vi "Move new property node.vi"(8 "error in":errorcluster, 9 "New objects created":refnum<vi>[](array[refnum]), 10 "Property Node Ref":refnum<vi>, 11 "Terminal Data Cluster":T1) -> (0 "error out":errorcluster)   [LabVIEW 2023]
doc: "Because a bundler will expand to the right once its labels are set, and we want to place the bundler to the left of a sink terminal, this VI will adjust the new objects created (a bundler and optional constant) to be posisioned the correct offset from the affected terminal. Offset is by default -15px.\n\nThis is not needed for bundlers on source terminals, so we ignore those."
panel:
  out "Move":i32
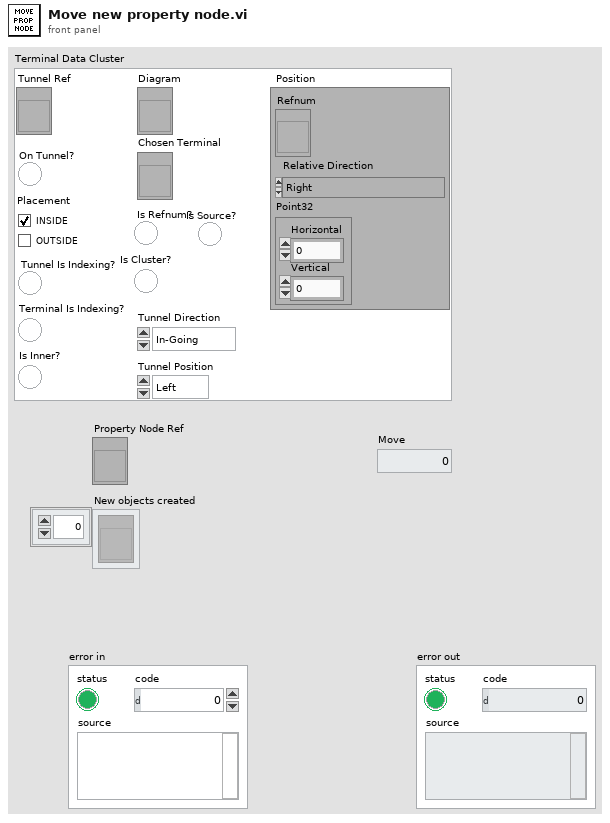
[diagram p1: front panel]
types:
  T1 = cluster{"Tunnel Ref":refnum<vi>, "On Tunnel?":bool, "Placement":enum32{"Choice 1", "Choice 2"}, "Tunnel Is Indexing?":bool, "Diagram":refnum<vi>, "Position":cluster{"Refnum":refnum<vi>, "Relative Direction":enum32{"Right", "Left", "Top", "Bottom", "Top Right", "Top Left", "Bottom Right", "Bottom Left"}, "Point32":cluster{"Horizontal":i32, "Vertical":i32}}, "Chosen Terminal":refnum<vi>, "Is Refnum?":bool, "Is Cluster?":bool, "Is Source?":bool, "Tunnel Direction":enum16{"In-Going", "Out-Going"}, "Tunnel Position":enum16{"Left", "Top", "Right", "Bottom"}, "Is Inner?":bool, "Terminal Is Indexing?":bool}
  T2 = typedef "LVRectTypeDef.ctl" = cluster{"Left":i16, "Top":i16, "Right":i16, "Bottom":i16}
  T3 = typedef "LVPositionTypeDef.ctl" = cluster{"Left":i32, "Top":i32}
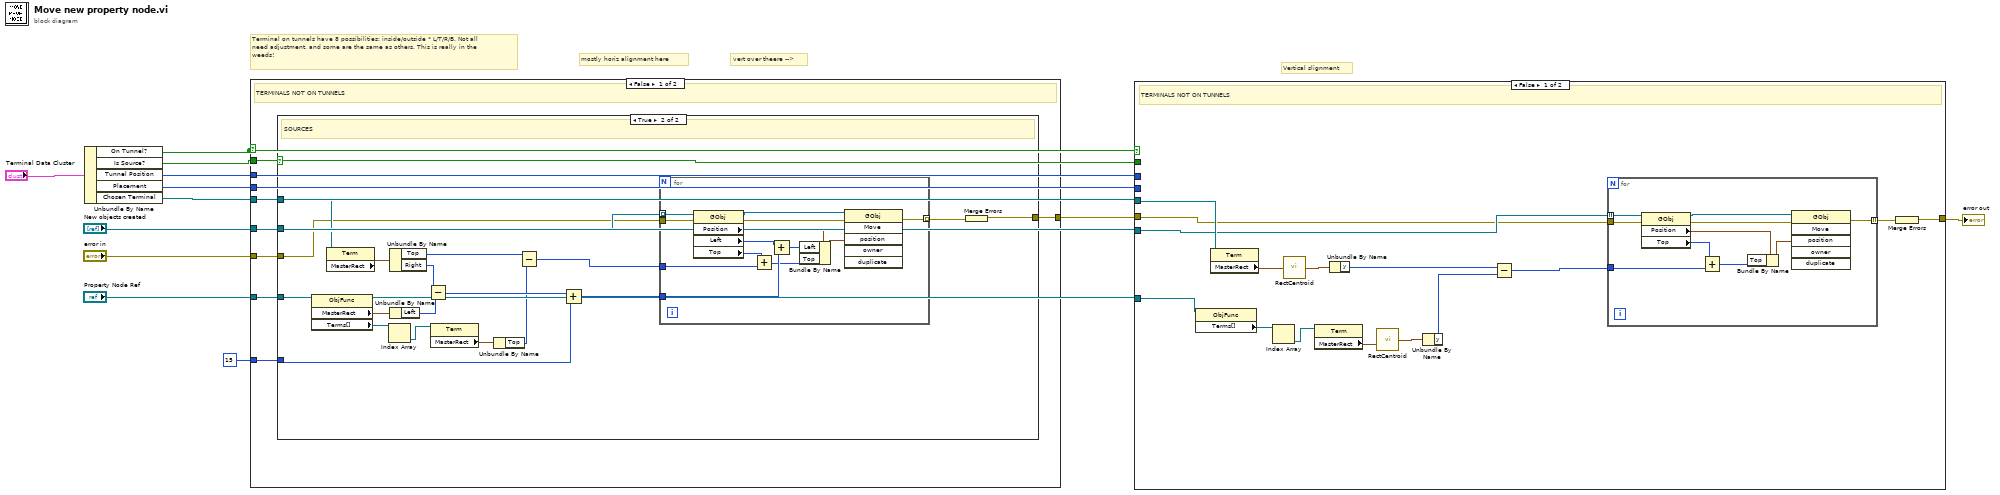
[diagram p0: block diagram]
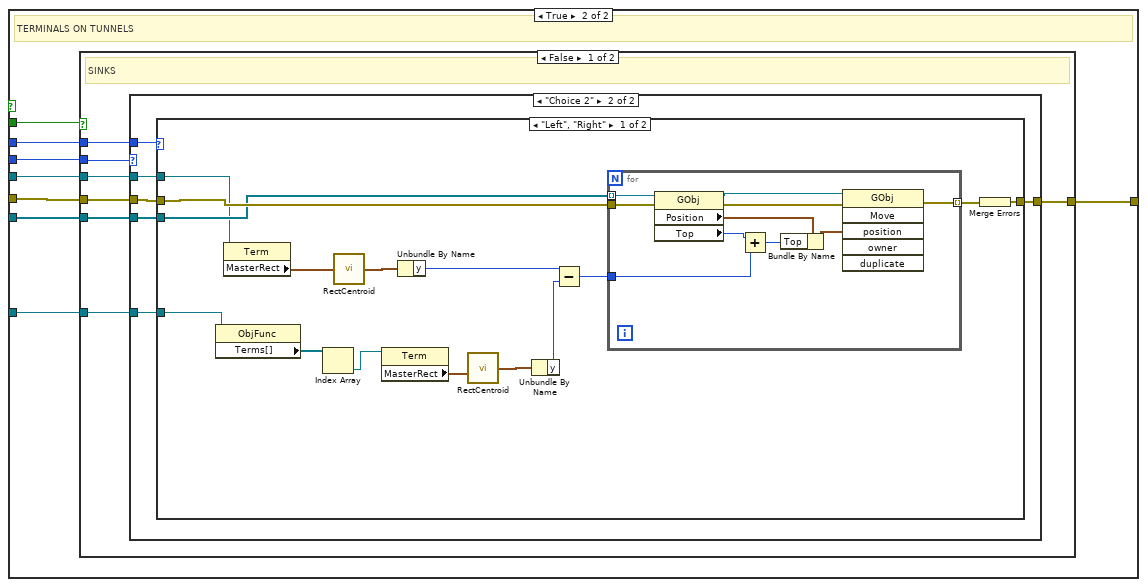
[diagram p2: hidden frame]
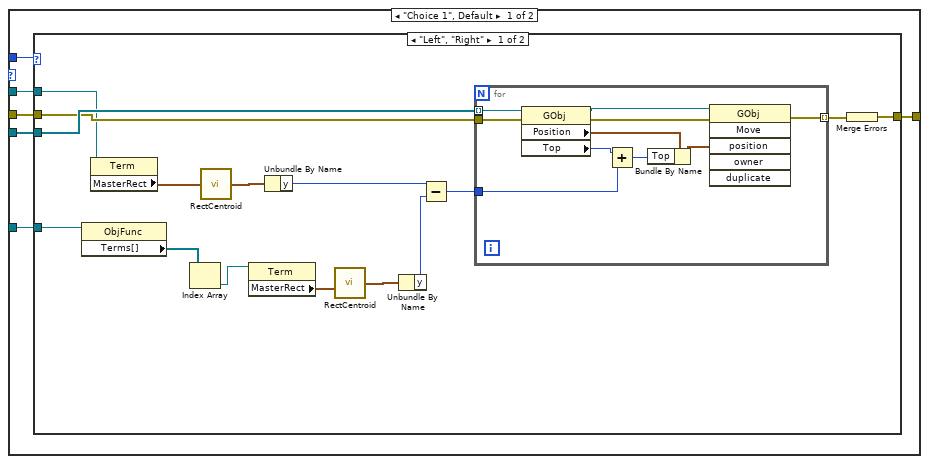
[diagram p3: hidden frame]
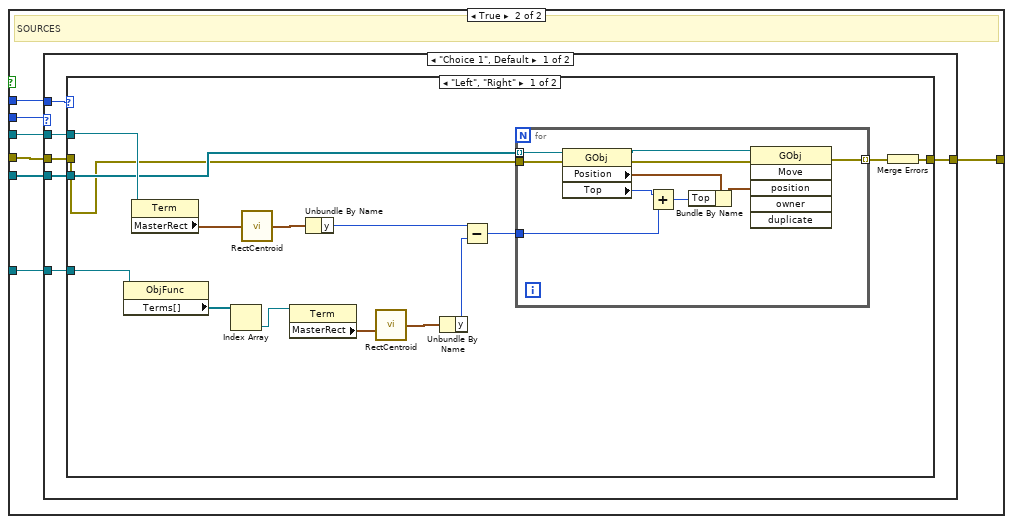
[diagram p6: hidden frame]
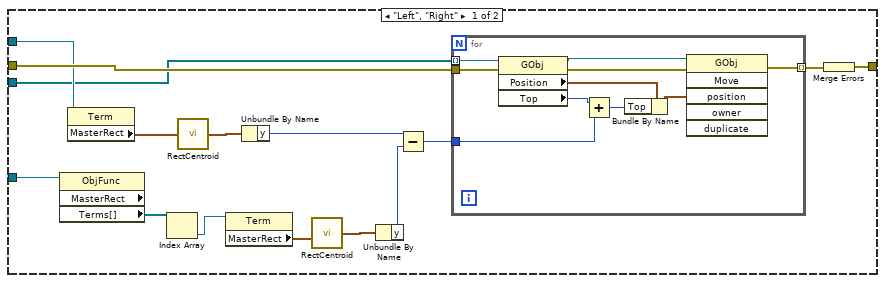
[diagram p9: hidden frame]
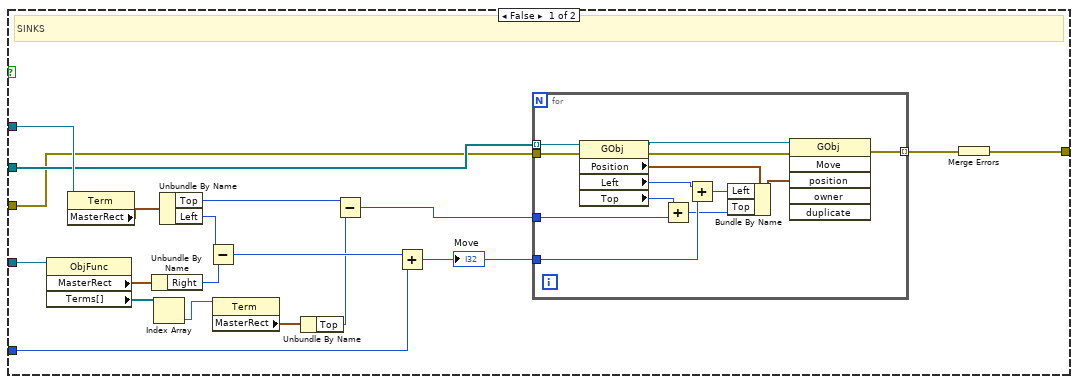
[diagram p10: hidden frame]
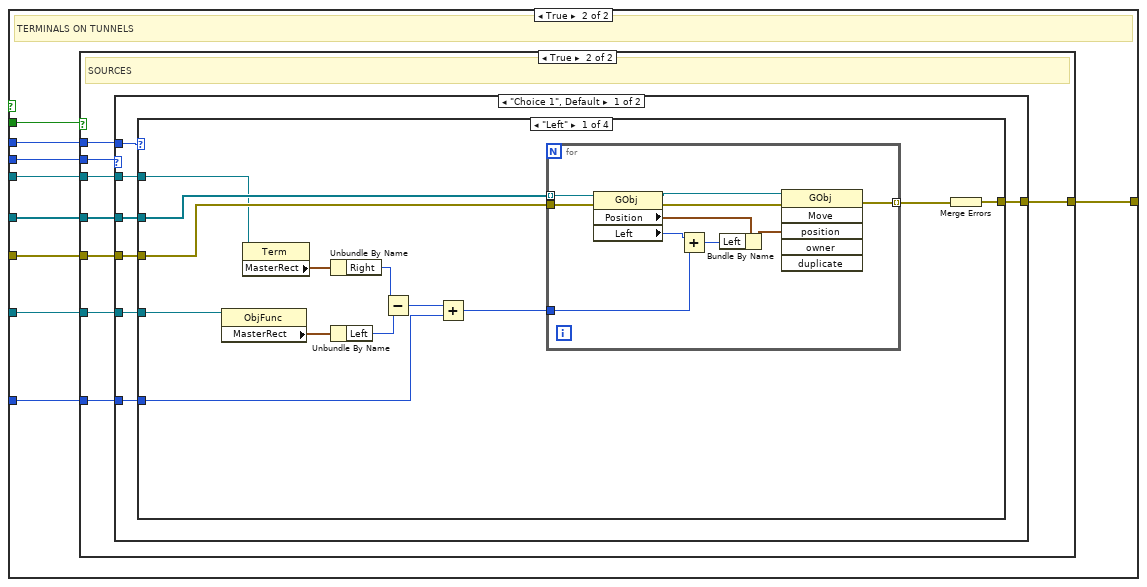
[diagram p11: hidden frame]
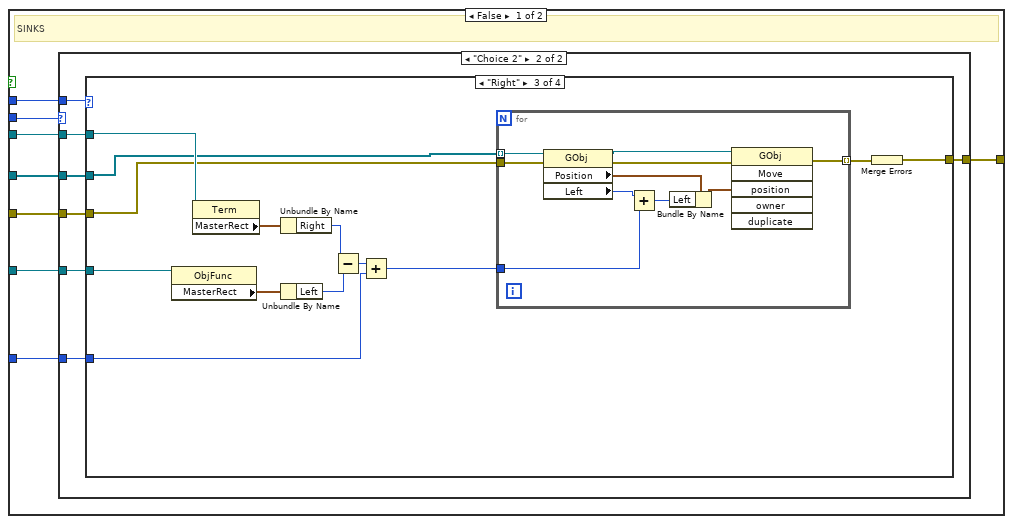
[diagram p12: hidden frame]
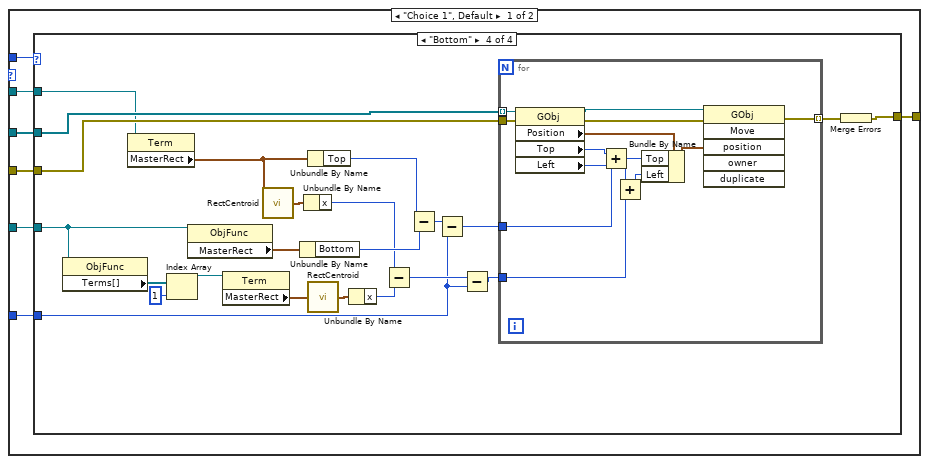
[diagram p13: hidden frame]
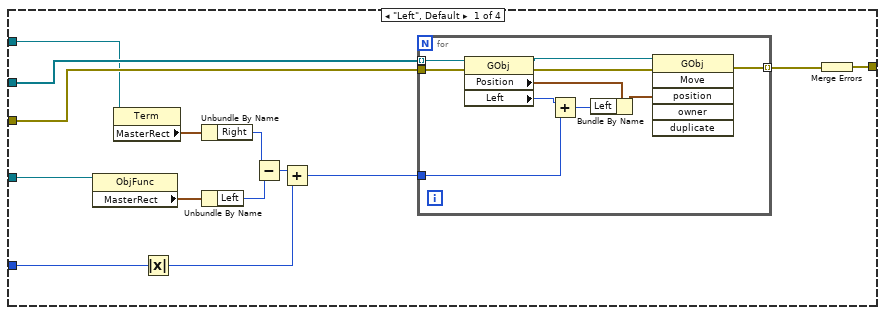
[diagram p14: hidden frame]
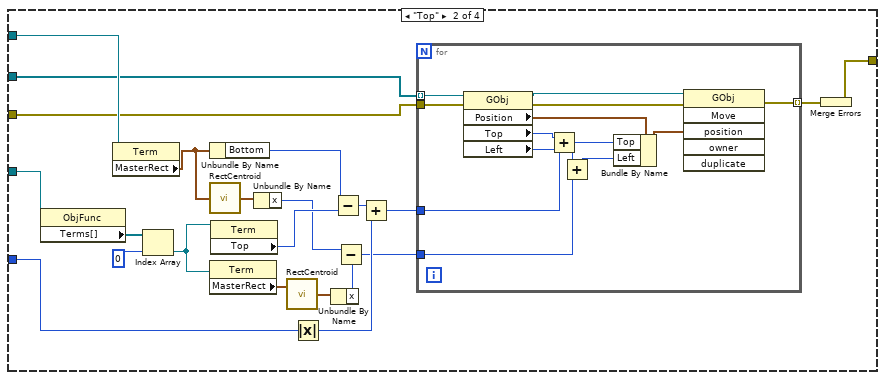
[diagram p15: hidden frame]
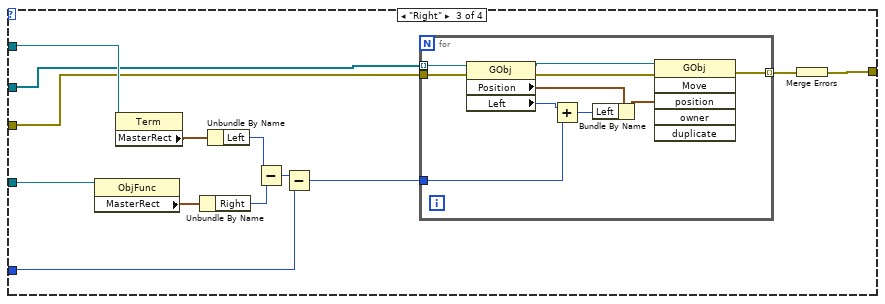
[diagram p16: hidden frame]
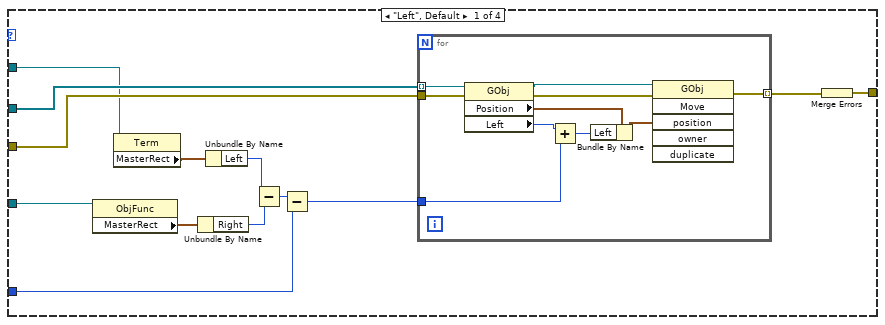
[diagram p17: hidden frame]
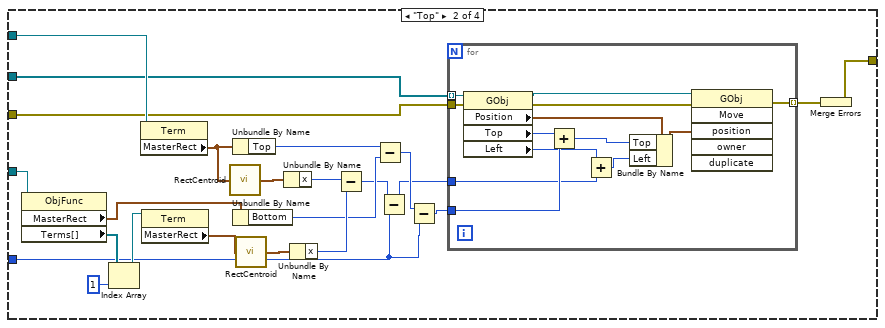
[diagram p18: hidden frame]
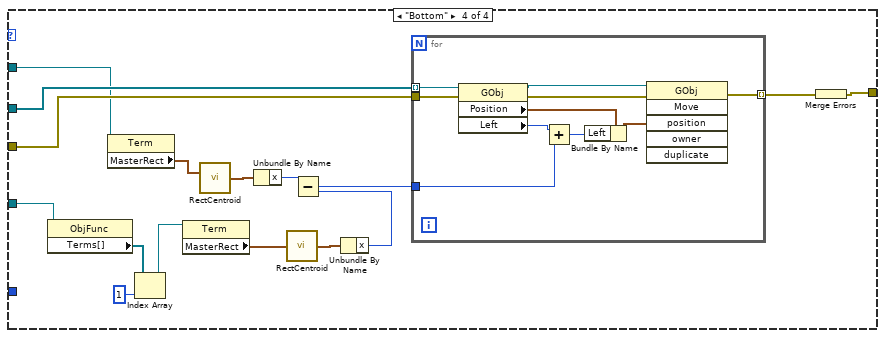
[diagram p19: hidden frame]
diagram:
  # "vert over theere -->"
  # "mostly horiz alignment here"
  # "Vertical slignment"
  # "Terminal on tunnels have 8 possibilities: inside/outside * L/T/R/B. Not all need adjustment, and some are the same as others. This is really in the weeds!"
  n1 = Unbundle By Name("Terminal Data Cluster") -> ("On Tunnel?"=w7:bool, "Is Source?"=w10:bool, "Tunnel Position"=w6:enum16{"Left", "Top", "Right", "Bottom"}, "Placement"=w5:enum32{"Choice 1", "Choice 2"}, "Chosen Terminal"=w4:refnum<vi>)
  n2 = case shown="False" w7 {
    tunnel: 15 ("Offset") -> [w13 w84]
    tunnel: "Property Node Ref" -> [w14 w86]
    tunnel: [w19 w89] -> w9
    tunnel: "error in" -> [w17 w88]
    tunnel: w10 -> [w18 w92]
    tunnel: w4 -> [w16 w85]
    tunnel: w6 -> [_ w91]
    tunnel: w5 -> [_ w90]
    tunnel: "New objects created" -> [w15 w87]
    frame False {
      # "TERMINALS NOT ON TUNNELS"
      n3 = case shown="True" w18 {
        tunnel: w13 -> [w37 w53]
        tunnel: w14 -> [w36 w54]
        tunnel: w16 -> [w34 w55]
        tunnel: [w28 w57] -> w19
        tunnel: w15 -> [w27 w56]
        tunnel: w17 -> [w26 w52]
        frame False {
          # "SINKS"
          n4 = property class="ObjFunc"(reference=w36) -> ("MasterRect"=w35:T2, "Terms[]"=w25:refnum<vi>[])  [unwired: 1 in, 2 out]
          n5 = property class="Term"(reference=w34) -> ("MasterRect"=w33:T2)  [unwired: 1 in, 2 out]
          n6 = Unbundle By Name(w35) -> ("Right"=w31:i16)
          n7 = Index Array(array=w25) -> (element=w24:refnum<vi>)  [unwired: 1 in]
          n8 = Unbundle By Name(w33) -> ("Top"=w22:i16, "Left"=w32:i16)
          n9 = Subtract(x=w32, y=w31) -> (x-y=w38:i16)
          n10 = property class="Term"(reference=w24) -> ("MasterRect"=w23:T2)  [unwired: 1 in, 2 out]
          n11 = Unbundle By Name(w23) -> ("Top"=w21:i16)
          n12 = Subtract(x=w22, y=w21) -> (x-y=w20:i16)
          n13 = Add(x=w38, y=w37) -> (x+y=w30:i32)
          "Move" <- w30
          n14 = for {
            tunnel: w27 -> [w51] mode=indexing
            tunnel: w30 -> [w48]
            tunnel: w26 -> [w44]
            tunnel: [w42] -> w29 mode=indexing
            tunnel: w20 -> [w40]
            n15 = property class="GObj"(reference=w51, error in=w44) -> (reference out=w50:refnum<vi>, error out=w43:errorcluster, "Position"=w47:T3, "Left"=w49:i32, "Top"=w41:i32)
            n16 = Add(x=w41, y=w40) -> (x+y=w39:i32)
            n17 = Add(x=w49, y=w48) -> (x+y=w46:i32)
            n18 = Bundle By Name(cluster=w47, "Left"=w46, "Top"=w39) -> (w45:T3)
            n19 = invoke class="GObj" method="Move"(reference=w50, error in=w43, "position"=w45) -> (error out=w42:errorcluster)  [unwired: 3 in, 5 out]
          }
          n20 = Merge Errors(w29) -> (w28:errorcluster)
        }
        frame True {
          # "SOURCES"
          n21 = property class="ObjFunc"(reference=w54) -> ("MasterRect"=w69:T2, "Terms[]"=w63:refnum<vi>[])  [unwired: 1 in, 2 out]
          n22 = property class="Term"(reference=w55) -> ("MasterRect"=w68:T2)  [unwired: 1 in, 2 out]
          n23 = Index Array(array=w63) -> (element=w62:refnum<vi>)  [unwired: 1 in]
          n24 = Unbundle By Name(w68) -> ("Top"=w60:i16, "Right"=w67:i16)
          n25 = Unbundle By Name(w69) -> ("Left"=w66:i16)
          n26 = Subtract(x=w67, y=w66) -> (x-y=w70:i16)
          n27 = property class="Term"(reference=w62) -> ("MasterRect"=w61:T2)  [unwired: 1 in, 2 out]
          n28 = Unbundle By Name(w61) -> ("Top"=w59:i16)
          n29 = Subtract(x=w60, y=w59) -> (x-y=w58:i16)
          n30 = Add(x=w70, y=w53) -> (x+y=w65:i32)
          n31 = for {
            tunnel: w56 -> [w83] mode=indexing
            tunnel: w65 -> [w80]
            tunnel: w52 -> [w76]
            tunnel: [w74] -> w64 mode=indexing
            tunnel: w58 -> [w72]
            n32 = property class="GObj"(reference=w83, error in=w76) -> (reference out=w82:refnum<vi>, error out=w75:errorcluster, "Position"=w79:T3, "Left"=w81:i32, "Top"=w73:i32)
            n33 = Add(x=w73, y=w72) -> (x+y=w71:i32)
            n34 = Add(x=w81, y=w80) -> (x+y=w78:i32)
            n35 = Bundle By Name(cluster=w79, "Left"=w78, "Top"=w71) -> (w77:T3)
            n36 = invoke class="GObj" method="Move"(reference=w82, error in=w75, "position"=w77) -> (error out=w74:errorcluster)  [unwired: 3 in, 5 out]
          }
          n37 = Merge Errors(w64) -> (w57:errorcluster)
        }
      }
    }
    frame True {
      # "TERMINALS ON TUNNELS"
      n38 = case shown="True" w92 {
        tunnel: w91 -> [w100 w348]
        tunnel: w90 -> [w99 w347]
        tunnel: [w98 w341] -> w89
        tunnel: w88 -> [w97 w344]
        tunnel: w87 -> [w96 w345]
        tunnel: w86 -> [w95 w343]
        tunnel: w85 -> [w94 w346]
        tunnel: w84 -> [w93 w342]
        frame False {
          # "SINKS"
          n39 = case shown="\"Choice 2\"" w99 {
            tunnel: w100 -> [w107 w232]
            tunnel: [w101 w231] -> w98
            tunnel: w97 -> [w104 w230]
            tunnel: w96 -> [w105 w229]
            tunnel: w95 -> [w102 w228]
            tunnel: w94 -> [w106 w227]
            tunnel: w93 -> [w103 w226]
            frame "Choice 1", Default {
              n40 = case shown="\"Bottom\"" w107 {
                tunnel: [w116 w147 w179 w203] -> w101
                tunnel: w104 -> [w120 w149 w176 w205]
                tunnel: w105 -> [w121 w148 w177 w206]
                tunnel: w102 -> [w119 w146 w175 w202]
                tunnel: w106 -> [w118 w150 w178 w204]
                tunnel: w103 -> [w117 w142 w174 w192]
                frame "Left", Default {
                  n41 = property class="ObjFunc"(reference=w119) -> ("MasterRect"=w114:T2)  [unwired: 1 in, 2 out]
                  n42 = property class="Term"(reference=w118) -> ("MasterRect"=w113:T2)  [unwired: 1 in, 2 out]
                  n43 = Absolute Value(x=w117) -> (abs(x)=w108:i32)
                  n44 = Unbundle By Name(w113) -> ("Right"=w112:i16)
                  n45 = Unbundle By Name(w114) -> ("Left"=w111:i16)
                  n46 = Subtract(x=w112, y=w111) -> (x-y=w115:i16)
                  n47 = Add(x=w115, y=w108) -> (x+y=w110:i32)
                  n48 = for {
                    tunnel: w110 -> [w129]
                    tunnel: [w124] -> w109 mode=indexing
                    tunnel: w121 -> [w123] mode=indexing
                    tunnel: w120 -> [w122]
                    n49 = property class="GObj"(reference=w123, error in=w122) -> (reference out=w131:refnum<vi>, error out=w125:errorcluster, "Position"=w128:T3, "Left"=w130:i32)
                    n50 = Add(x=w130, y=w129) -> (x+y=w127:i32)
                    n51 = Bundle By Name(cluster=w128, "Left"=w127) -> (w126:T3)
                    n52 = invoke class="GObj" method="Move"(reference=w131, error in=w125, "position"=w126) -> (error out=w124:errorcluster)  [unwired: 3 in, 5 out]
                  }
                  n53 = Merge Errors(w109) -> (w116:errorcluster)
                }
                frame "Top" {
                  n54 = property class="ObjFunc"(reference=w146) -> ("Terms[]"=w145:refnum<vi>[])  [unwired: 1 in, 2 out]
                  n55 = property class="Term"(reference=w150) -> ("MasterRect"=w137:T2)  [unwired: 1 in, 2 out]
                  n56 = Index Array(array=w145, index=0) -> (element=w138:refnum<vi>)
                  n57 = Unbundle By Name(w137) -> ("Bottom"=w140:i16)
                  n58 = call <vilib>:"RectCentroid.vi"("rect"=w137) -> ("point"=w136:cluster{"x":i16, "y":i16})
                  n59 = property class="Term"(reference=w138) -> ("MasterRect"=w133:T2)  [unwired: 1 in, 2 out]
                  n60 = property class="Term"(reference=w138) -> ("Top"=w144:i32)  [unwired: 1 in, 2 out]
                  n61 = Unbundle By Name(w136) -> ("x"=w135:i16)
                  n62 = call <vilib>:"RectCentroid.vi"("rect"=w133) -> ("point"=w134:cluster{"x":i16, "y":i16})
                  n63 = Absolute Value(x=w142) -> (abs(x)=w143:i32)
                  n64 = Unbundle By Name(w134) -> ("x"=w132:i16)
                  n65 = Subtract(x=w140, y=w144) -> (x-y=w153:i32)
                  n66 = Subtract(x=w135, y=w132) -> (x-y=w141:i16)
                  n67 = Add(x=w153, y=w143) -> (x+y=w152:i32)
                  n68 = for {
                    tunnel: w152 -> [w164]
                    tunnel: [w159] -> w151 mode=indexing
                    tunnel: w149 -> [w158]
                    tunnel: w148 -> [w157] mode=indexing
                    tunnel: w141 -> [w155]
                    n69 = property class="GObj"(reference=w157, error in=w158) -> (reference out=w166:refnum<vi>, error out=w160:errorcluster, "Position"=w163:T3, "Top"=w165:i32, "Left"=w156:i32)
                    n70 = Add(x=w165, y=w164) -> (x+y=w162:i32)
                    n71 = Add(x=w156, y=w155) -> (x+y=w154:i32)
                    n72 = Bundle By Name(cluster=w163, "Top"=w162, "Left"=w154) -> (w161:T3)
                    n73 = invoke class="GObj" method="Move"(reference=w166, error in=w160, "position"=w161) -> (error out=w159:errorcluster)  [unwired: 3 in, 5 out]
                  }
                  n74 = Merge Errors(w151) -> (w147:errorcluster)
                }
                frame "Right" {
                  n75 = property class="ObjFunc"(reference=w175) -> ("MasterRect"=w172:T2)  [unwired: 1 in, 2 out]
                  n76 = property class="Term"(reference=w178) -> ("MasterRect"=w171:T2)  [unwired: 1 in, 2 out]
                  n77 = Unbundle By Name(w172) -> ("Right"=w169:i16)
                  n78 = Unbundle By Name(w171) -> ("Left"=w170:i16)
                  n79 = Subtract(x=w170, y=w169) -> (x-y=w173:i16)
                  n80 = Subtract(x=w173, y=w174) -> (x-y=w168:i32)
                  n81 = for {
                    tunnel: w177 -> [w189] mode=indexing
                    tunnel: w168 -> [w186]
                    tunnel: w176 -> [w182]
                    tunnel: [w180] -> w167 mode=indexing
                    n82 = property class="GObj"(reference=w189, error in=w182) -> (reference out=w188:refnum<vi>, error out=w181:errorcluster, "Position"=w185:T3, "Left"=w187:i32)
                    n83 = Add(x=w187, y=w186) -> (x+y=w184:i32)
                    n84 = Bundle By Name(cluster=w185, "Left"=w184) -> (w183:T3)
                    n85 = invoke class="GObj" method="Move"(reference=w188, error in=w181, "position"=w183) -> (error out=w180:errorcluster)  [unwired: 3 in, 5 out]
                  }
                  n86 = Merge Errors(w167) -> (w179:errorcluster)
                }
                frame "Bottom" {
                  n87 = property class="ObjFunc"(reference=w202) -> ("Terms[]"=w201:refnum<vi>[])  [unwired: 1 in, 2 out]
                  n88 = property class="Term"(reference=w204) -> ("MasterRect"=w195:T2)  [unwired: 1 in, 2 out]
                  n89 = Index Array(array=w201, index=1) -> (element=w200:refnum<vi>)
                  n90 = property class="ObjFunc"(reference=w202) -> ("MasterRect"=w211:T2)  [unwired: 1 in, 2 out]
                  n91 = property class="Term"(reference=w200) -> ("MasterRect"=w199:T2)  [unwired: 1 in, 2 out]
                  n92 = call <vilib>:"RectCentroid.vi"("rect"=w195) -> ("point"=w196:cluster{"x":i16, "y":i16})
                  n93 = Unbundle By Name(w211) -> ("Bottom"=w209:i16)
                  n94 = Unbundle By Name(w196) -> ("x"=w194:i16)
                  n95 = Unbundle By Name(w195) -> ("Top"=w210:i16)
                  n96 = call <vilib>:"RectCentroid.vi"("rect"=w199) -> ("point"=w198:cluster{"x":i16, "y":i16})
                  n97 = Unbundle By Name(w198) -> ("x"=w197:i16)
                  n98 = Subtract(x=w194, y=w197) -> (x-y=w193:i16)
                  n99 = Subtract(x=w210, y=w209) -> (x-y=w212:i16)
                  n100 = Subtract(x=w212, y=w192) -> (x-y=w208:i32)
                  n101 = Subtract(x=w193, y=w192) -> (x-y=w191:i32)
                  n102 = for {
                    tunnel: w206 -> [w225] mode=indexing
                    tunnel: w208 -> [w222]
                    tunnel: w205 -> [w218]
                    tunnel: [w216] -> w207 mode=indexing
                    tunnel: w191 -> [w214]
                    n103 = property class="GObj"(reference=w225, error in=w218) -> (reference out=w224:refnum<vi>, error out=w217:errorcluster, "Position"=w221:T3, "Top"=w223:i32, "Left"=w215:i32)
                    n104 = Add(x=w223, y=w222) -> (x+y=w220:i32)
                    n105 = Add(x=w215, y=w214) -> (x+y=w213:i32)
                    n106 = Bundle By Name(cluster=w221, "Top"=w220, "Left"=w213) -> (w219:T3)
                    n107 = invoke class="GObj" method="Move"(reference=w224, error in=w217, "position"=w219) -> (error out=w216:errorcluster)  [unwired: 3 in, 5 out]
                  }
                  n108 = Merge Errors(w207) -> (w203:errorcluster)
                }
              }
            }
            frame "Choice 2" {
              n109 = case shown="\"Right\"" w232 {
                tunnel: [w233 w273 w304 w326] -> w231
                tunnel: w230 -> [w237 w275 w301 w328]
                tunnel: w229 -> [w238 w274 w302 w329]
                tunnel: w228 -> [w236 w264 w300 w318]
                tunnel: w227 -> [w235 w276 w303 w327]
                tunnel: w226 -> [w234 w259 w299 _]
                frame "Left", Default {
                  n110 = property class="ObjFunc"(reference=w236) -> ("MasterRect"=w244:T2)  [unwired: 1 in, 2 out]
                  n111 = property class="Term"(reference=w235) -> ("MasterRect"=w243:T2)  [unwired: 1 in, 2 out]
                  n112 = Unbundle By Name(w244) -> ("Right"=w241:i16)
                  n113 = Unbundle By Name(w243) -> ("Left"=w242:i16)
                  n114 = Subtract(x=w242, y=w241) -> (x-y=w245:i16)
                  n115 = Subtract(x=w245, y=w234) -> (x-y=w240:i32)
                  n116 = for {
                    tunnel: w240 -> [w253]
                    tunnel: [w248] -> w239 mode=indexing
                    tunnel: w238 -> [w247] mode=indexing
                    tunnel: w237 -> [w246]
                    n117 = property class="GObj"(reference=w247, error in=w246) -> (reference out=w255:refnum<vi>, error out=w249:errorcluster, "Position"=w252:T3, "Left"=w254:i32)
                    n118 = Add(x=w254, y=w253) -> (x+y=w251:i32)
                    n119 = Bundle By Name(cluster=w252, "Left"=w251) -> (w250:T3)
                    n120 = invoke class="GObj" method="Move"(reference=w255, error in=w249, "position"=w250) -> (error out=w248:errorcluster)  [unwired: 3 in, 5 out]
                  }
                  n121 = Merge Errors(w239) -> (w233:errorcluster)
                }
                frame "Top" {
                  n122 = property class="ObjFunc"(reference=w264) -> ("MasterRect"=w257:T2, "Terms[]"=w267:refnum<vi>[])  [unwired: 1 in, 2 out]
                  n123 = Index Array(array=w267, index=1) -> (element=w265:refnum<vi>)
                  n124 = property class="Term"(reference=w276) -> ("MasterRect"=w271:T2)  [unwired: 1 in, 2 out]
                  n125 = property class="Term"(reference=w265) -> ("MasterRect"=w256:T2)  [unwired: 1 in, 2 out]
                  n126 = call <vilib>:"RectCentroid.vi"("rect"=w271) -> ("point"=w272:cluster{"x":i16, "y":i16})
                  n127 = Unbundle By Name(w271) -> ("Top"=w278:i16)
                  n128 = Unbundle By Name(w257) -> ("Bottom"=w263:i16)
                  n129 = call <vilib>:"RectCentroid.vi"("rect"=w256) -> ("point"=w270:cluster{"x":i16, "y":i16})
                  n130 = Unbundle By Name(w272) -> ("x"=w269:i16)
                  n131 = Unbundle By Name(w270) -> ("x"=w268:i16)
                  n132 = Subtract(x=w269, y=w268) -> (x-y=w260:i16)
                  n133 = Subtract(x=w278, y=w263) -> (x-y=w262:i16)
                  n134 = Subtract(x=w260, y=w259) -> (x-y=w258:i32)
                  n135 = Subtract(x=w262, y=w259) -> (x-y=w261:i32)
                  n136 = for {
                    tunnel: w261 -> [w289]
                    tunnel: [w284] -> w277 mode=indexing
                    tunnel: w275 -> [w283]
                    tunnel: w274 -> [w282] mode=indexing
                    tunnel: w258 -> [w279]
                    n137 = property class="GObj"(reference=w282, error in=w283) -> (reference out=w291:refnum<vi>, error out=w285:errorcluster, "Position"=w288:T3, "Top"=w290:i32, "Left"=w281:i32)
                    n138 = Add(x=w290, y=w289) -> (x+y=w287:i32)
                    n139 = Add(x=w281, y=w279) -> (x+y=w280:i32)
                    n140 = Bundle By Name(cluster=w288, "Top"=w287, "Left"=w280) -> (w286:T3)
                    n141 = invoke class="GObj" method="Move"(reference=w291, error in=w285, "position"=w286) -> (error out=w284:errorcluster)  [unwired: 3 in, 5 out]
                  }
                  n142 = Merge Errors(w277) -> (w273:errorcluster)
                }
                frame "Right" {
                  n143 = property class="ObjFunc"(reference=w300) -> ("MasterRect"=w297:T2)  [unwired: 1 in, 2 out]
                  n144 = property class="Term"(reference=w303) -> ("MasterRect"=w296:T2)  [unwired: 1 in, 2 out]
                  n145 = Unbundle By Name(w296) -> ("Right"=w295:i16)
                  n146 = Unbundle By Name(w297) -> ("Left"=w294:i16)
                  n147 = Subtract(x=w295, y=w294) -> (x-y=w298:i16)
                  n148 = Add(x=w298, y=w299) -> (x+y=w293:i32)
                  n149 = for {
                    tunnel: w302 -> [w314] mode=indexing
                    tunnel: w293 -> [w311]
                    tunnel: w301 -> [w307]
                    tunnel: [w305] -> w292 mode=indexing
                    n150 = property class="GObj"(reference=w314, error in=w307) -> (reference out=w313:refnum<vi>, error out=w306:errorcluster, "Position"=w310:T3, "Left"=w312:i32)
                    n151 = Add(x=w312, y=w311) -> (x+y=w309:i32)
                    n152 = Bundle By Name(cluster=w310, "Left"=w309) -> (w308:T3)
                    n153 = invoke class="GObj" method="Move"(reference=w313, error in=w306, "position"=w308) -> (error out=w305:errorcluster)  [unwired: 3 in, 5 out]
                  }
                  n154 = Merge Errors(w292) -> (w304:errorcluster)
                }
                frame "Bottom" {
                  n155 = property class="ObjFunc"(reference=w318) -> ("Terms[]"=w317:refnum<vi>[])  [unwired: 1 in, 2 out]
                  n156 = property class="Term"(reference=w327) -> ("MasterRect"=w322:T2)  [unwired: 1 in, 2 out]
                  n157 = Index Array(array=w317, index=1) -> (element=w315:refnum<vi>)
                  n158 = property class="Term"(reference=w315) -> ("MasterRect"=w323:T2)  [unwired: 1 in, 2 out]
                  n159 = call <vilib>:"RectCentroid.vi"("rect"=w322) -> ("point"=w325:cluster{"x":i16, "y":i16})
                  n160 = Unbundle By Name(w325) -> ("x"=w321:i16)
                  n161 = call <vilib>:"RectCentroid.vi"("rect"=w323) -> ("point"=w324:cluster{"x":i16, "y":i16})
                  n162 = Unbundle By Name(w324) -> ("x"=w320:i16)
                  n163 = Subtract(x=w321, y=w320) -> (x-y=w319:i16)
                  n164 = for {
                    tunnel: w329 -> [w340] mode=indexing
                    tunnel: w328 -> [w334]
                    tunnel: [w332] -> w330 mode=indexing
                    tunnel: w319 -> [w331]
                    n165 = property class="GObj"(reference=w340, error in=w334) -> (reference out=w339:refnum<vi>, error out=w333:errorcluster, "Position"=w337:T3, "Left"=w338:i32)
                    n166 = Add(x=w338, y=w331) -> (x+y=w336:i32)
                    n167 = Bundle By Name(cluster=w337, "Left"=w336) -> (w335:T3)
                    n168 = invoke class="GObj" method="Move"(reference=w339, error in=w333, "position"=w335) -> (error out=w332:errorcluster)  [unwired: 3 in, 5 out]
                  }
                  n169 = Merge Errors(w330) -> (w326:errorcluster)
                }
              }
            }
          }
        }
        frame True {
          # "SOURCES"
          n170 = case shown="\"Choice 1\", Default" w347 {
            tunnel: w348 -> [w355 w442]
            tunnel: w346 -> [w354 w441]
            tunnel: w345 -> [w353 w440]
            tunnel: w344 -> [w352 w439]
            tunnel: w343 -> [w351 w438]
            tunnel: w342 -> [w350 w437]
            tunnel: [w349 w436] -> w341
            frame "Choice 1", Default {
              n171 = case shown="\"Left\"" w355 {
                tunnel: [w363 w379 w392 w412] -> w349
                tunnel: w352 -> [w367 w379 w389 w414]
                tunnel: w353 -> [w368 _ w390 w415]
                tunnel: w351 -> [w366 _ w388 w411]
                tunnel: w354 -> [w365 _ w391 w413]
                tunnel: w350 -> [w364 _ w387 w404]
                frame "Left" {
                  n172 = property class="ObjFunc"(reference=w366) -> ("MasterRect"=w361:T2)  [unwired: 1 in, 2 out]
                  n173 = property class="Term"(reference=w365) -> ("MasterRect"=w360:T2)  [unwired: 1 in, 2 out]
                  n174 = Unbundle By Name(w360) -> ("Right"=w359:i16)
                  n175 = Unbundle By Name(w361) -> ("Left"=w358:i16)
                  n176 = Subtract(x=w359, y=w358) -> (x-y=w362:i16)
                  n177 = Add(x=w362, y=w364) -> (x+y=w357:i32)
                  n178 = for {
                    tunnel: w357 -> [w376]
                    tunnel: [w371] -> w356 mode=indexing
                    tunnel: w368 -> [w370] mode=indexing
                    tunnel: w367 -> [w369]
                    n179 = property class="GObj"(reference=w370, error in=w369) -> (reference out=w378:refnum<vi>, error out=w372:errorcluster, "Position"=w375:T3, "Left"=w377:i32)
                    n180 = Add(x=w377, y=w376) -> (x+y=w374:i32)
                    n181 = Bundle By Name(cluster=w375, "Left"=w374) -> (w373:T3)
                    n182 = invoke class="GObj" method="Move"(reference=w378, error in=w372, "position"=w373) -> (error out=w371:errorcluster)  [unwired: 3 in, 5 out]
                  }
                  n183 = Merge Errors(w356) -> (w363:errorcluster)
                }
                frame Default {
                }
                frame "Right" {
                  n184 = property class="ObjFunc"(reference=w388) -> ("MasterRect"=w385:T2)  [unwired: 1 in, 2 out]
                  n185 = property class="Term"(reference=w391) -> ("MasterRect"=w384:T2)  [unwired: 1 in, 2 out]
                  n186 = Unbundle By Name(w385) -> ("Right"=w382:i16)
                  n187 = Unbundle By Name(w384) -> ("Left"=w383:i16)
                  n188 = Subtract(x=w383, y=w382) -> (x-y=w386:i16)
                  n189 = Subtract(x=w386, y=w387) -> (x-y=w381:i32)
                  n190 = for {
                    tunnel: w390 -> [w402] mode=indexing
                    tunnel: w381 -> [w399]
                    tunnel: w389 -> [w395]
                    tunnel: [w393] -> w380 mode=indexing
                    n191 = property class="GObj"(reference=w402, error in=w395) -> (reference out=w401:refnum<vi>, error out=w394:errorcluster, "Position"=w398:T3, "Left"=w400:i32)
                    n192 = Add(x=w400, y=w399) -> (x+y=w397:i32)
                    n193 = Bundle By Name(cluster=w398, "Left"=w397) -> (w396:T3)
                    n194 = invoke class="GObj" method="Move"(reference=w401, error in=w394, "position"=w396) -> (error out=w393:errorcluster)  [unwired: 3 in, 5 out]
                  }
                  n195 = Merge Errors(w380) -> (w392:errorcluster)
                }
                frame "Bottom" {
                  n196 = property class="ObjFunc"(reference=w411) -> ("Terms[]"=w410:refnum<vi>[])  [unwired: 1 in, 2 out]
                  n197 = property class="Term"(reference=w413) -> ("MasterRect"=w420:T2)  [unwired: 1 in, 2 out]
                  n198 = property class="ObjFunc"(reference=w411) -> ("MasterRect"=w421:T2)  [unwired: 1 in, 2 out]
                  n199 = Index Array(array=w410, index=0) -> (element=w408:refnum<vi>)
                  n200 = Unbundle By Name(w420) -> ("Top"=w419:i16, "Left"=w407:i16)
                  n201 = property class="Term"(reference=w408) -> ("Left"=w406:i32)  [unwired: 1 in, 2 out]
                  n202 = Unbundle By Name(w421) -> ("Bottom"=w418:i16)
                  n203 = Subtract(x=w419, y=w418) -> (x-y=w422:i16)
                  n204 = Subtract(x=w407, y=w406) -> (x-y=w405:i32)
                  n205 = Subtract(x=w422, y=w404) -> (x-y=w417:i32)
                  n206 = Add(x=w405, y=w404) -> (x+y=w403:i32)
                  n207 = for {
                    tunnel: w415 -> [w435] mode=indexing
                    tunnel: w417 -> [w432]
                    tunnel: w414 -> [w428]
                    tunnel: [w426] -> w416 mode=indexing
                    tunnel: w403 -> [w423]
                    n208 = property class="GObj"(reference=w435, error in=w428) -> (reference out=w434:refnum<vi>, error out=w427:errorcluster, "Position"=w431:T3, "Top"=w433:i32, "Left"=w425:i32)
                    n209 = Add(x=w433, y=w432) -> (x+y=w430:i32)
                    n210 = Add(x=w425, y=w423) -> (x+y=w424:i32)
                    n211 = Bundle By Name(cluster=w431, "Top"=w430, "Left"=w424) -> (w429:T3)
                    n212 = invoke class="GObj" method="Move"(reference=w434, error in=w427, "position"=w429) -> (error out=w426:errorcluster)  [unwired: 3 in, 5 out]
                  }
                  n213 = Merge Errors(w416) -> (w412:errorcluster)
                }
              }
            }
            frame "Choice 2" {
              n214 = case shown="\"Left\", Default" w442 {
                tunnel: [w443 w482 w520 w547] -> w436
                tunnel: w439 -> [w447 w481 w518 w544]
                tunnel: w440 -> [w448 w479 w516 w545]
                tunnel: w438 -> [w446 w474 w519 w543]
                tunnel: w441 -> [w445 w480 w517 w546]
                tunnel: w437 -> [w444 w467 w502 w542]
                frame "Left", Default {
                  n215 = property class="ObjFunc"(reference=w446) -> ("MasterRect"=w454:T2)  [unwired: 1 in, 2 out]
                  n216 = property class="Term"(reference=w445) -> ("MasterRect"=w453:T2)  [unwired: 1 in, 2 out]
                  n217 = Unbundle By Name(w454) -> ("Right"=w451:i16)
                  n218 = Unbundle By Name(w453) -> ("Left"=w452:i16)
                  n219 = Subtract(x=w452, y=w451) -> (x-y=w455:i16)
                  n220 = Subtract(x=w455, y=w444) -> (x-y=w450:i32)
                  n221 = for {
                    tunnel: w450 -> [w463]
                    tunnel: [w458] -> w449 mode=indexing
                    tunnel: w448 -> [w457] mode=indexing
                    tunnel: w447 -> [w456]
                    n222 = property class="GObj"(reference=w457, error in=w456) -> (reference out=w465:refnum<vi>, error out=w459:errorcluster, "Position"=w462:T3, "Left"=w464:i32)
                    n223 = Add(x=w464, y=w463) -> (x+y=w461:i32)
                    n224 = Bundle By Name(cluster=w462, "Left"=w461) -> (w460:T3)
                    n225 = invoke class="GObj" method="Move"(reference=w465, error in=w459, "position"=w460) -> (error out=w458:errorcluster)  [unwired: 3 in, 5 out]
                  }
                  n226 = Merge Errors(w449) -> (w443:errorcluster)
                }
                frame "Top" {
                  n227 = property class="ObjFunc"(reference=w474) -> ("Terms[]"=w473:refnum<vi>[])  [unwired: 1 in, 2 out]
                  n228 = property class="ObjFunc"(reference=w474) -> ("MasterRect"=w476:T2)  [unwired: 1 in, 2 out]
                  n229 = property class="Term"(reference=w480) -> ("MasterRect"=w484:T2)  [unwired: 1 in, 2 out]
                  n230 = Index Array(array=w473, index=0) -> (element=w471:refnum<vi>)
                  n231 = property class="Term"(reference=w471) -> ("Left"=w469:i32)  [unwired: 1 in, 2 out]
                  n232 = Unbundle By Name(w476) -> ("Bottom"=w475:i16)
                  n233 = Unbundle By Name(w484) -> ("Top"=w483:i16, "Right"=w470:i16)
                  n234 = Subtract(x=w470, y=w469) -> (x-y=w468:i32)
                  n235 = Subtract(x=w483, y=w475) -> (x-y=w485:i16)
                  n236 = Subtract(x=w485, y=w467) -> (x-y=w477:i32)
                  n237 = Add(x=w468, y=w467) -> (x+y=w466:i32)
                  n238 = for {
                    tunnel: w481 -> [w492]
                    tunnel: w479 -> [w491] mode=indexing
                    tunnel: [w490] -> w478 mode=indexing
                    tunnel: w477 -> [w489]
                    tunnel: w466 -> [w486]
                    n239 = property class="GObj"(reference=w491, error in=w492) -> (reference out=w498:refnum<vi>, error out=w493:errorcluster, "Position"=w496:T3, "Top"=w497:i32, "Left"=w488:i32)
                    n240 = Add(x=w497, y=w489) -> (x+y=w495:i32)
                    n241 = Add(x=w488, y=w486) -> (x+y=w487:i32)
                    n242 = Bundle By Name(cluster=w496, "Top"=w495, "Left"=w487) -> (w494:T3)
                    n243 = invoke class="GObj" method="Move"(reference=w498, error in=w493, "position"=w494) -> (error out=w490:errorcluster)  [unwired: 3 in, 5 out]
                  }
                  n244 = Merge Errors(w478) -> (w482:errorcluster)
                }
                frame "Bottom" {
                  # "corrrrects weird issue that only happens in this case"
                  n245 = property class="ObjFunc"(reference=w519) -> ("Terms[]"=w514:refnum<vi>[])  [unwired: 1 in, 2 out]
                  n246 = property class="Term"(reference=w517) -> ("MasterRect"=w506:T2)  [unwired: 1 in, 2 out]
                  n247 = Index Array(array=w514, index=0) -> (element=w511:refnum<vi>)
                  n248 = Unbundle By Name(w506) -> ("Bottom"=w500:i16)
                  n249 = property class="Term"(reference=w511) -> ("MasterRect"=w505:T2)  [unwired: 1 in, 2 out]
                  n250 = call <vilib>:"RectCentroid.vi"("rect"=w506) -> ("point"=w509:cluster{"x":i16, "y":i16})
                  n251 = Absolute Value(x=w502) -> (abs(x)=w499:i32)
                  n252 = Unbundle By Name(w509) -> ("x"=w508:i16)
                  n253 = Unbundle By Name(w505) -> ("Top"=w504:i16)
                  n254 = call <vilib>:"RectCentroid.vi"("rect"=w505) -> ("point"=w512:cluster{"x":i16, "y":i16})
                  n255 = Unbundle By Name(w512) -> ("x"=w510:i16)
                  n256 = Subtract(x=w500, y=w504) -> (x-y=w503:i16)
                  n257 = Add(x=w503, y=w499) -> (x+y=w501:i32)
                  n258 = Subtract(x=w508, y=w510) -> (x-y=w507:i16)
                  n259 = for {
                    tunnel: w518 -> [w528]
                    tunnel: w516 -> [w527] mode=indexing
                    tunnel: [w526] -> w515 mode=indexing
                    tunnel: w507 -> [w525]
                    tunnel: w501 -> [w522]
                    n260 = property class="GObj"(reference=w527, error in=w528) -> (reference out=w534:refnum<vi>, error out=w529:errorcluster, "Position"=w532:T3, "Left"=w533:i32, "Top"=w524:i32)
                    n261 = Decrement(x=w525) -> (x-1=w521:i16)
                    n262 = Add(x=w533, y=w521) -> (x+y=w531:i32)
                    n263 = Add(x=w524, y=w522) -> (x+y=w523:i32)
                    n264 = Bundle By Name(cluster=w532, "Left"=w531, "Top"=w523) -> (w530:T3)
                    n265 = invoke class="GObj" method="Move"(reference=w534, error in=w529, "position"=w530) -> (error out=w526:errorcluster)  [unwired: 3 in, 5 out]
                  }
                  n266 = Merge Errors(w515) -> (w520:errorcluster)
                }
                frame "Right" {
                  n267 = property class="ObjFunc"(reference=w543) -> ("MasterRect"=w540:T2)  [unwired: 1 in, 2 out]
                  n268 = property class="Term"(reference=w546) -> ("MasterRect"=w539:T2)  [unwired: 1 in, 2 out]
                  n269 = Unbundle By Name(w539) -> ("Right"=w538:i16)
                  n270 = Unbundle By Name(w540) -> ("Left"=w537:i16)
                  n271 = Subtract(x=w538, y=w537) -> (x-y=w541:i16)
                  n272 = Add(x=w541, y=w542) -> (x+y=w536:i32)
                  n273 = for {
                    tunnel: w545 -> [w557] mode=indexing
                    tunnel: w536 -> [w554]
                    tunnel: w544 -> [w550]
                    tunnel: [w548] -> w535 mode=indexing
                    n274 = property class="GObj"(reference=w557, error in=w550) -> (reference out=w556:refnum<vi>, error out=w549:errorcluster, "Position"=w553:T3, "Left"=w555:i32)
                    n275 = Add(x=w555, y=w554) -> (x+y=w552:i32)
                    n276 = Bundle By Name(cluster=w553, "Left"=w552) -> (w551:T3)
                    n277 = invoke class="GObj" method="Move"(reference=w556, error in=w549, "position"=w551) -> (error out=w548:errorcluster)  [unwired: 3 in, 5 out]
                  }
                  n278 = Merge Errors(w535) -> (w547:errorcluster)
                }
              }
            }
          }
        }
      }
    }
  }
  n279 = case shown="False" w7 {
    tunnel: "Property Node Ref" -> [w572 w584]
    tunnel: [w571 w587] -> w8
    tunnel: w9 -> [w568 w586]
    tunnel: w10 -> [_ w590]
    tunnel: w4 -> [w570 w583]
    tunnel: w6 -> [_ w589]
    tunnel: w5 -> [_ w588]
    tunnel: "New objects created" -> [w569 w585]
    frame False {
      # "TERMINALS NOT ON TUNNELS"
      n280 = property class="ObjFunc"(reference=w572) -> ("Terms[]"=w566:refnum<vi>[])  [unwired: 1 in, 2 out]
      n281 = property class="Term"(reference=w570) -> ("MasterRect"=w563:T2)  [unwired: 1 in, 2 out]
      n282 = Index Array(array=w566) -> (element=w565:refnum<vi>)  [unwired: 1 in]
      n283 = call <vilib>:"RectCentroid.vi"("rect"=w563) -> ("point"=w562:cluster{"x":i16, "y":i16})
      n284 = property class="Term"(reference=w565) -> ("MasterRect"=w559:T2)  [unwired: 1 in, 2 out]
      n285 = Unbundle By Name(w562) -> ("y"=w561:i16)
      n286 = call <vilib>:"RectCentroid.vi"("rect"=w559) -> ("point"=w560:cluster{"x":i16, "y":i16})
      n287 = Unbundle By Name(w560) -> ("y"=w558:i16)
      n288 = Subtract(x=w561, y=w558) -> (x-y=w564:i16)
      n289 = for {
        tunnel: w569 -> [w582] mode=indexing
        tunnel: w568 -> [w578]
        tunnel: [w576] -> w567 mode=indexing
        tunnel: w564 -> [w574]
        n290 = property class="GObj"(reference=w582, error in=w578) -> (reference out=w581:refnum<vi>, error out=w577:errorcluster, "Position"=w580:T3, "Top"=w575:i32)
        n291 = Add(x=w575, y=w574) -> (x+y=w573:i32)
        n292 = Bundle By Name(cluster=w580, "Top"=w573) -> (w579:T3)
        n293 = invoke class="GObj" method="Move"(reference=w581, error in=w577, "position"=w579) -> (error out=w576:errorcluster)  [unwired: 3 in, 5 out]
      }
      n294 = Merge Errors(w567) -> (w571:errorcluster)
    }
    frame True {
      # "TERMINALS ON TUNNELS"
      n295 = case shown="False" w590 {
        tunnel: w589 -> [w597 w668]
        tunnel: w588 -> [w596 w667]
        tunnel: [w595 w662] -> w587
        tunnel: w586 -> [w594 w664]
        tunnel: w585 -> [w593 w665]
        tunnel: w584 -> [w592 w663]
        tunnel: w583 -> [w591 w666]
        frame False {
          # "SINKS"
          n296 = case shown="\"Choice 2\"" w596 {
            tunnel: w597 -> [w603 w635]
            tunnel: [w598 w634] -> w595
            tunnel: w594 -> [w600 w633]
            tunnel: w593 -> [w601 w632]
            tunnel: w592 -> [w599 w631]
            tunnel: w591 -> [w602 w630]
            frame "Choice 1", Default {
              n297 = case shown="\"Left\", \"Right\"" w603 {
                tunnel: [w615 w629] -> w598
                tunnel: w600 -> [w617 w629]
                tunnel: w601 -> [w618 _]
                tunnel: w599 -> [w607 _]
                tunnel: w602 -> [w616 _]
                frame "Left", "Right" {
                  n298 = property class="ObjFunc"(reference=w607) -> ("Terms[]"=w608:refnum<vi>[])  [unwired: 1 in, 2 out]
                  n299 = property class="Term"(reference=w616) -> ("MasterRect"=w612:T2)  [unwired: 1 in, 2 out]
                  n300 = Index Array(array=w608) -> (element=w609:refnum<vi>)  [unwired: 1 in]
                  n301 = call <vilib>:"RectCentroid.vi"("rect"=w612) -> ("point"=w613:cluster{"x":i16, "y":i16})
                  n302 = property class="Term"(reference=w609) -> ("MasterRect"=w611:T2)  [unwired: 1 in, 2 out]
                  n303 = Unbundle By Name(w613) -> ("y"=w606:i16)
                  n304 = call <vilib>:"RectCentroid.vi"("rect"=w611) -> ("point"=w610:cluster{"x":i16, "y":i16})
                  n305 = Unbundle By Name(w610) -> ("y"=w605:i16)
                  n306 = Subtract(x=w606, y=w605) -> (x-y=w604:i16)
                  n307 = for {
                    tunnel: [w622] -> w614 mode=indexing
                    tunnel: w618 -> [w621] mode=indexing
                    tunnel: w617 -> [w620]
                    tunnel: w604 -> [w619]
                    n308 = property class="GObj"(reference=w621, error in=w620) -> (reference out=w628:refnum<vi>, error out=w623:errorcluster, "Position"=w626:T3, "Top"=w627:i32)
                    n309 = Add(x=w627, y=w619) -> (x+y=w625:i32)
                    n310 = Bundle By Name(cluster=w626, "Top"=w625) -> (w624:T3)
                    n311 = invoke class="GObj" method="Move"(reference=w628, error in=w623, "position"=w624) -> (error out=w622:errorcluster)  [unwired: 3 in, 5 out]
                  }
                  n312 = Merge Errors(w614) -> (w615:errorcluster)
                }
                frame Default {
                }
              }
            }
            frame "Choice 2" {
              n313 = case shown="\"Left\", \"Right\"" w635 {
                tunnel: [w640 w661] -> w634
                tunnel: w633 -> [w639 w661]
                tunnel: w632 -> [w638 _]
                tunnel: w631 -> [w636 _]
                tunnel: w630 -> [w637 _]
                frame "Left", "Right" {
                  n314 = property class="ObjFunc"(reference=w636) -> ("Terms[]"=w644:refnum<vi>[])  [unwired: 1 in, 2 out]
                  n315 = property class="Term"(reference=w637) -> ("MasterRect"=w648:T2)  [unwired: 1 in, 2 out]
                  n316 = Index Array(array=w644) -> (element=w645:refnum<vi>)  [unwired: 1 in]
                  n317 = call <vilib>:"RectCentroid.vi"("rect"=w648) -> ("point"=w649:cluster{"x":i16, "y":i16})
                  n318 = property class="Term"(reference=w645) -> ("MasterRect"=w647:T2)  [unwired: 1 in, 2 out]
                  n319 = Unbundle By Name(w649) -> ("y"=w643:i16)
                  n320 = call <vilib>:"RectCentroid.vi"("rect"=w647) -> ("point"=w646:cluster{"x":i16, "y":i16})
                  n321 = Unbundle By Name(w646) -> ("y"=w642:i16)
                  n322 = Subtract(x=w643, y=w642) -> (x-y=w641:i16)
                  n323 = for {
                    tunnel: [w654] -> w650 mode=indexing
                    tunnel: w638 -> [w653] mode=indexing
                    tunnel: w639 -> [w652]
                    tunnel: w641 -> [w651]
                    n324 = property class="GObj"(reference=w653, error in=w652) -> (reference out=w660:refnum<vi>, error out=w655:errorcluster, "Position"=w658:T3, "Top"=w659:i32)
                    n325 = Add(x=w659, y=w651) -> (x+y=w657:i32)
                    n326 = Bundle By Name(cluster=w658, "Top"=w657) -> (w656:T3)
                    n327 = invoke class="GObj" method="Move"(reference=w660, error in=w655, "position"=w656) -> (error out=w654:errorcluster)  [unwired: 3 in, 5 out]
                  }
                  n328 = Merge Errors(w650) -> (w640:errorcluster)
                }
                frame Default {
                }
              }
            }
          }
        }
        frame True {
          # "SOURCES"
          n329 = case shown="\"Choice 1\", Default" w667 {
            tunnel: w668 -> [w674 w706]
            tunnel: w666 -> [w673 w705]
            tunnel: w665 -> [w672 w704]
            tunnel: w664 -> [w671 w701]
            tunnel: w663 -> [w670 w703]
            tunnel: [w669 w702] -> w662
            frame "Choice 1", Default {
              n330 = case shown="\"Left\", \"Right\"" w674 {
                tunnel: [w676 w700] -> w669
                tunnel: w671 -> [w677 w700]
                tunnel: w672 -> [w678 _]
                tunnel: w670 -> [w675 _]
                tunnel: w673 -> [w679 _]
                frame "Left", "Right" {
                  n331 = property class="ObjFunc"(reference=w675) -> ("Terms[]"=w683:refnum<vi>[])  [unwired: 1 in, 2 out]
                  n332 = property class="Term"(reference=w679) -> ("MasterRect"=w687:T2)  [unwired: 1 in, 2 out]
                  n333 = Index Array(array=w683) -> (element=w684:refnum<vi>)  [unwired: 1 in]
                  n334 = call <vilib>:"RectCentroid.vi"("rect"=w687) -> ("point"=w688:cluster{"x":i16, "y":i16})
                  n335 = property class="Term"(reference=w684) -> ("MasterRect"=w686:T2)  [unwired: 1 in, 2 out]
                  n336 = Unbundle By Name(w688) -> ("y"=w682:i16)
                  n337 = call <vilib>:"RectCentroid.vi"("rect"=w686) -> ("point"=w685:cluster{"x":i16, "y":i16})
                  n338 = Unbundle By Name(w685) -> ("y"=w681:i16)
                  n339 = Subtract(x=w682, y=w681) -> (x-y=w680:i16)
                  n340 = for {
                    tunnel: [w693] -> w689 mode=indexing
                    tunnel: w678 -> [w692] mode=indexing
                    tunnel: w677 -> [w691]
                    tunnel: w680 -> [w690]
                    n341 = property class="GObj"(reference=w692, error in=w691) -> (reference out=w699:refnum<vi>, error out=w694:errorcluster, "Position"=w697:T3, "Top"=w698:i32)
                    n342 = Add(x=w698, y=w690) -> (x+y=w696:i32)
                    n343 = Bundle By Name(cluster=w697, "Top"=w696) -> (w695:T3)
                    n344 = invoke class="GObj" method="Move"(reference=w699, error in=w694, "position"=w695) -> (error out=w693:errorcluster)  [unwired: 3 in, 5 out]
                  }
                  n345 = Merge Errors(w689) -> (w676:errorcluster)
                }
                frame Default {
                }
              }
            }
            frame "Choice 2" {
              n346 = case shown="Default" w706 {
                tunnel: [w711 w732] -> w702
                tunnel: w704 -> [w707 _]
                tunnel: w703 -> [w708 _]
                tunnel: w705 -> [w709 _]
                tunnel: w701 -> [w710 w732]
                frame "Left", "Right" {
                  n347 = property class="ObjFunc" props=["MasterRect", "Terms[]"](reference=w708) -> ("Terms[]"=w715:refnum<vi>[])  [unwired: 1 in, 3 out]
                  n348 = property class="Term"(reference=w709) -> ("MasterRect"=w719:T2)  [unwired: 1 in, 2 out]
                  n349 = Index Array(array=w715) -> (element=w716:refnum<vi>)  [unwired: 1 in]
                  n350 = call <vilib>:"RectCentroid.vi"("rect"=w719) -> ("point"=w720:cluster{"x":i16, "y":i16})
                  n351 = property class="Term"(reference=w716) -> ("MasterRect"=w718:T2)  [unwired: 1 in, 2 out]
                  n352 = Unbundle By Name(w720) -> ("y"=w714:i16)
                  n353 = call <vilib>:"RectCentroid.vi"("rect"=w718) -> ("point"=w717:cluster{"x":i16, "y":i16})
                  n354 = Unbundle By Name(w717) -> ("y"=w713:i16)
                  n355 = Subtract(x=w714, y=w713) -> (x-y=w712:i16)
                  n356 = for {
                    tunnel: [w725] -> w721 mode=indexing
                    tunnel: w707 -> [w724] mode=indexing
                    tunnel: w710 -> [w723]
                    tunnel: w712 -> [w722]
                    n357 = property class="GObj"(reference=w724, error in=w723) -> (reference out=w731:refnum<vi>, error out=w726:errorcluster, "Position"=w729:T3, "Top"=w730:i32)
                    n358 = Add(x=w730, y=w722) -> (x+y=w728:i32)
                    n359 = Bundle By Name(cluster=w729, "Top"=w728) -> (w727:T3)
                    n360 = invoke class="GObj" method="Move"(reference=w731, error in=w726, "position"=w727) -> (error out=w725:errorcluster)  [unwired: 3 in, 5 out]
                  }
                  n361 = Merge Errors(w721) -> (w711:errorcluster)
                }
                frame Default {
                }
              }
            }
          }
        }
      }
    }
  }
  "error out" <- w8
